vi "Prune.vi"(8 "error in (no error)":errorcluster, 11 "FileAppender in":refnum<class "FileAppender.lvclass">) -> (0 "error out":errorcluster, 3 "FileAppender out":refnum<class "FileAppender.lvclass">)   [LabVIEW 2026, in "Lumberjack.lvlib" / "FileAppender.lvclass"]
uses:
  FileAppender.lvclass
  FileAppender.lvclass/FileAppender.ctl
  Lumberjack.lvlib
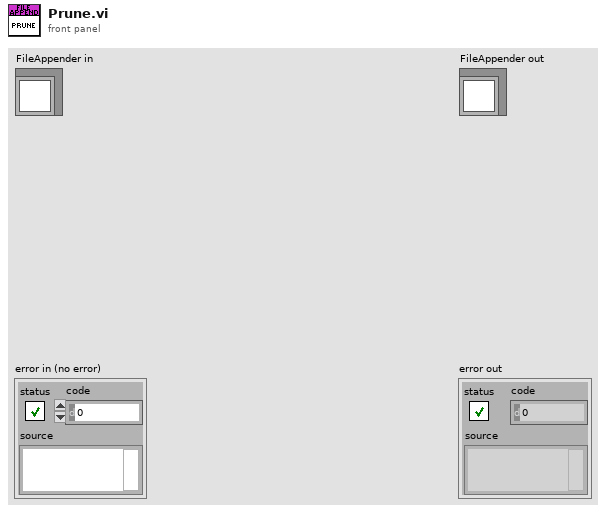
[diagram p1: front panel]
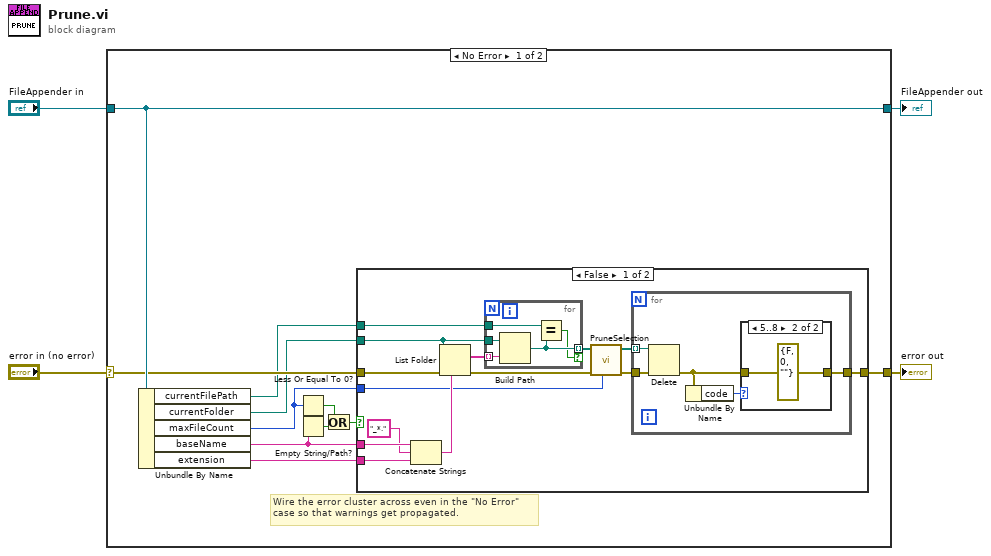
[diagram p0: block diagram]
diagram:
  n1 = case shown="No Error" "error in (no error)" {
    selector: "error in (no error)" -> [w14 w43]
    tunnel: [w13 w43] -> w3
    tunnel: [w15 w42] -> w1
    tunnel: "FileAppender in" -> [w15 w42]
    frame No Error {
      # "Wire the error cluster across even in the \"No Error\"\ncase so that warnings get propagated."
      n2 = Unbundle By Name(w15) -> ("currentFilePath"=w5:path, "currentFolder"=w6:path, "maxFileCount"=w9:i32, "baseName"=w11:string, "extension"=w10:string)
      n3 = Less Or Equal To 0?(x=w9) -> (x <= 0?=w8:bool)
      n4 = Empty String/Path?(string/path=w11) -> (empty?=w7:bool)
      n5 = Or(x=w8, y=w7) -> (x .or. y?=w12:bool)
      n6 = case shown="False" w12 {
        tunnel: w14 -> [w28 w41]
        tunnel: [w17 w41] -> w13
        tunnel: w6 -> [w20 _]
        tunnel: w9 -> [w22 _]
        tunnel: w11 -> [w26 _]
        tunnel: w10 -> [w24 _]
        tunnel: w5 -> [w19 _]
        frame False {
          n7 = Concatenate Strings(w26, "_*." ("string"), w24) -> (w23:string)
          n8 = List Folder(path=w20, pattern=w23, error in=w28) -> (filenames=w21:string[], error out=w27:errorcluster)  [unwired: 1 in, 2 out]
          n9 = for {
            tunnel: w21 -> [w40] mode=indexing
            tunnel: w20 -> [w39]
            tunnel: w19 -> [w38]
            tunnel: [w37] -> w18 mode=indexing if=w36
            n10 = Build Path(base path=w39, name or relative path=w40) -> (appended path=w37:path)
            n11 = Equal?(x=w38, y=w37) -> (x = y?=w36:bool)
          }
          n12 = call "PruneSelection.vi"("maxFileCount"=w22, "error in (no error)"=w27, "ExistingFiles"=w18) -> ("error out"=w17:errorcluster, "FilesToDelete"=w16:path[])  [unwired: 7 in]
          n13 = for {
            tunnel: w17 -> [w33]
            tunnel: w16 -> [w32] mode=indexing
            tunnel: [w29] -> _
            n14 = Delete(path (use dialog)=w32, error in=w33) -> (error out=w31:errorcluster)  [unwired: 3 in, 2 out]
            n15 = Unbundle By Name(w31) -> ("code"=w30:i32)
            n16 = case shown="5..8" w30 {
              tunnel: w31 -> [w34 _]
              tunnel: [w34 errorcluster {"status"=FALSE, "code"=0, "source"=""} ("error out")] -> w29
              frame Default {
              }
              frame 5..8 {
              }
            }
          }
        }
        frame True {
        }
      }
    }
    frame Error {
    }
  }
  "error out" <- w3
  "FileAppender out" <- w1
